vi "Get Base Class Name and Path.vi"(11 "Class":refnum<class>) -> (1 "Success?":bool, 2 "Class Path":path, 3 "Base Class Name":string)   [LabVIEW 2020, in "ClassLoader.lvlib"]
doc: "Get base class name (file name without extension) and path to the given class."
uses:
  ClassLoader.lvlib
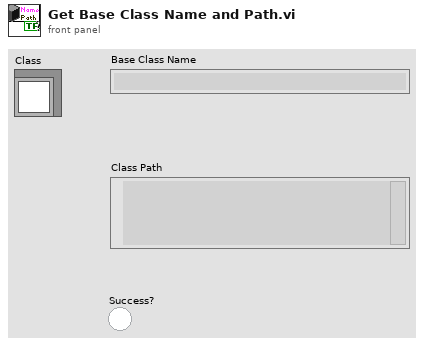
[diagram p1: front panel]
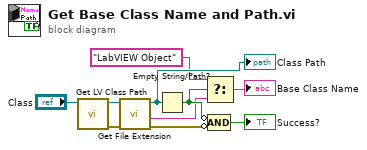
[diagram p0: block diagram]
diagram:
  n1 = call <vilib>:"Get LV Class Path.vi"("object"="Class") -> ("error out"=w10:errorcluster, "class path"=w9:path)  [unwired: 9 in]
  n2 = call <vilib>:"Get File Extension.vi"("error in (no error)"=w10, "file"=w9) -> ("error out"=w7:errorcluster, "filename without extension"=w3:string, "dup file"=w8:path)  [unwired: 5 in, 2 out]
  "Class Path" <- w8
  n3 = Empty String/Path?(string/path=w8) -> (empty?=w5:bool)
  n4 = Select(t="LabVIEW Object", s=w5, f=w3) -> (s? t:f=→"Base Class Name":string)
  n5 = Compound Arithmetic op=AND(invert w5, invert w7) -> (→"Success?":bool)
